vi "Get Reply.vi"(8 "error in (no error)":errorcluster, 10 "node address":u16 format="%.0x", 11 "masterHdl in":T2) -> (0 "error out":errorcluster, 1 "Cmd":T1 items=["NONE", "ROR", "ROL", "MST", "MVP", "SAP", "GAP", "STAP", "RSAP", "SGP", "GGP"], 2 "status":u8, 3 "master ref out":T2, 4 "value":i32, 5 "raw data":u8[](array[numeric]), 6 "module adr":u8, 7 "reply addr":u8)   [LabVIEW 2017, in "NI_Robotics_KUKA youBot Host.lvlib"]
uses:
  <vilib>/robotics/KUKA youBot/NI_Robotics_KUKA youBot Host.lvlib
  <vilib>/robotics/KUKA youBot/EtherCAT/LowLevel/Mater Handler.ctl
  <vilib>/robotics/KUKA youBot/EtherCAT/CmdCtrls/Param Cmd.ctl
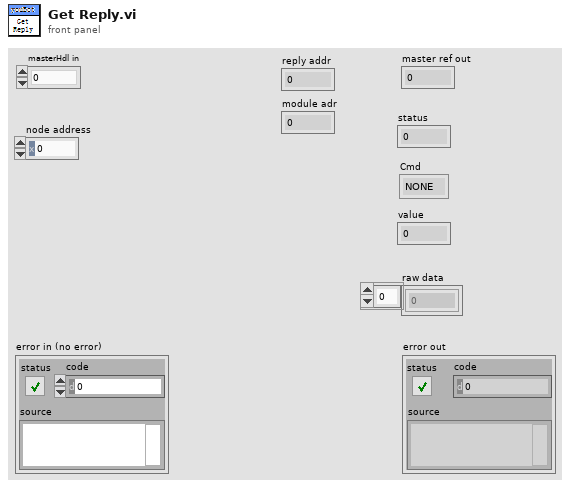
[diagram p1: front panel]
types:
  T1 = typedef "NI_Robotics_KUKA youBot Host.lvlib/Param Cmd.ctl" = u8
  T2 = typedef "NI_Robotics_KUKA youBot Host.lvlib/Mater Handler.ctl" = i32
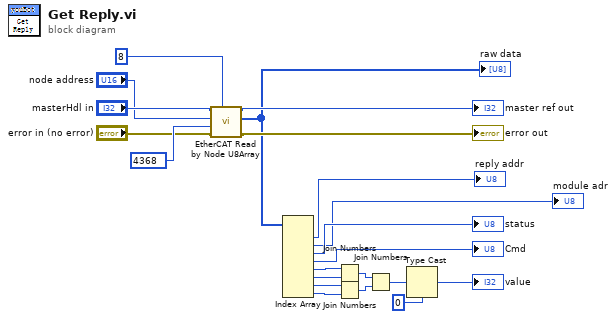
[diagram p0: block diagram]
diagram:
  n1 = call <vilib>:"EtherCAT Read by Node U8Array.vi"("dataLen"=u32 8, "error in (no error)"="error in (no error)", "startAddr"=u16 4368, "nodeAddr"="node address", "masterHdl in"="masterHdl in") -> ("error out"=→"error out":errorcluster, "data"=w1:u8[], "masterHdl out"=→"master ref out":T2)  [unwired: 4 in]
  "raw data" <- w1
  n2 = Index Array(array=w1) -> (element #1=→"reply addr":u8, element #2=→"module adr":u8, element #3=→"status":u8, element #4=→"Cmd":u8, element #5=w15:u8, element #6=w16:u8, element #7=w17:u8, element #8=w18:u8)  [unwired: 8 in]
  n3 = Join Numbers(hi=w15, lo=w16) -> ((hi.lo)=w19:u16)
  n4 = Join Numbers(hi=w17, lo=w18) -> ((hi.lo)=w20:u16)
  n5 = Join Numbers(hi=w19, lo=w20) -> ((hi.lo)=w21:u32)
  n6 = Type Cast(type=0 ("(hi.lo)"), x=w21) -> (*(type *) &x=→"value":i32)
